vi "Execute Single Statement (String Parameters).vi"(6 "Oids":i32[](array[numeric]), 8 "error in (no error)":errorcluster, 9 "Parameters":string[](array[string]), 10 "SQL (Single Command)":string, 11 "PQ Connection in":refnum<class "PQ Connection.lvclass">) -> (0 "error out":errorcluster, 1 "First Result with Rows returned":refnum<class "PQ Result.lvclass">, 2 "Number of Rows":i32, 3 "PQ Connection out":refnum<class "PQ Connection.lvclass">)   [LabVIEW 2013, in "PQ Connection.lvclass"]
uses:
  PQ Connection.lvclass
  Result/PQ Result.lvclass
  PQ Connection.lvclass/PQ Connection.ctl
  Result/PQ Result.lvclass/PQ Result.ctl
  Support/PQ Support.lvlib
  libpq.dll
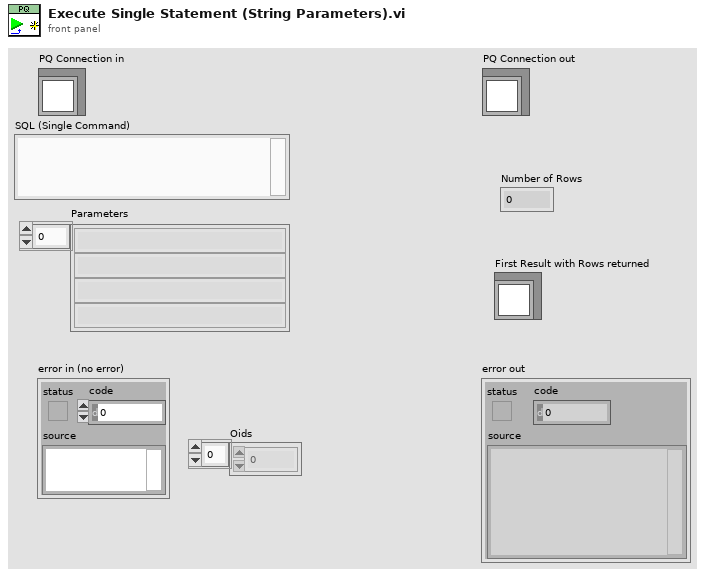
[diagram p1: front panel]
types:
  T1 = typedef "PQ Result.lvclass/Result Status.ctl" = enum32{"PGRES_EMPTY_QUERY", "PGRES_COMMAND_OK", "PGRES_TUPLES_OK", "PGRES_COPY_OUT", "PGRES_COPY_IN", "PGRES_BAD_RESPONSE", "PGRES_NONFATAL_ERROR", "PGRES_FATAL_ERROR", "PGRES_COPY_BOTH", "PGRES_SINGLE_TUPLE"}
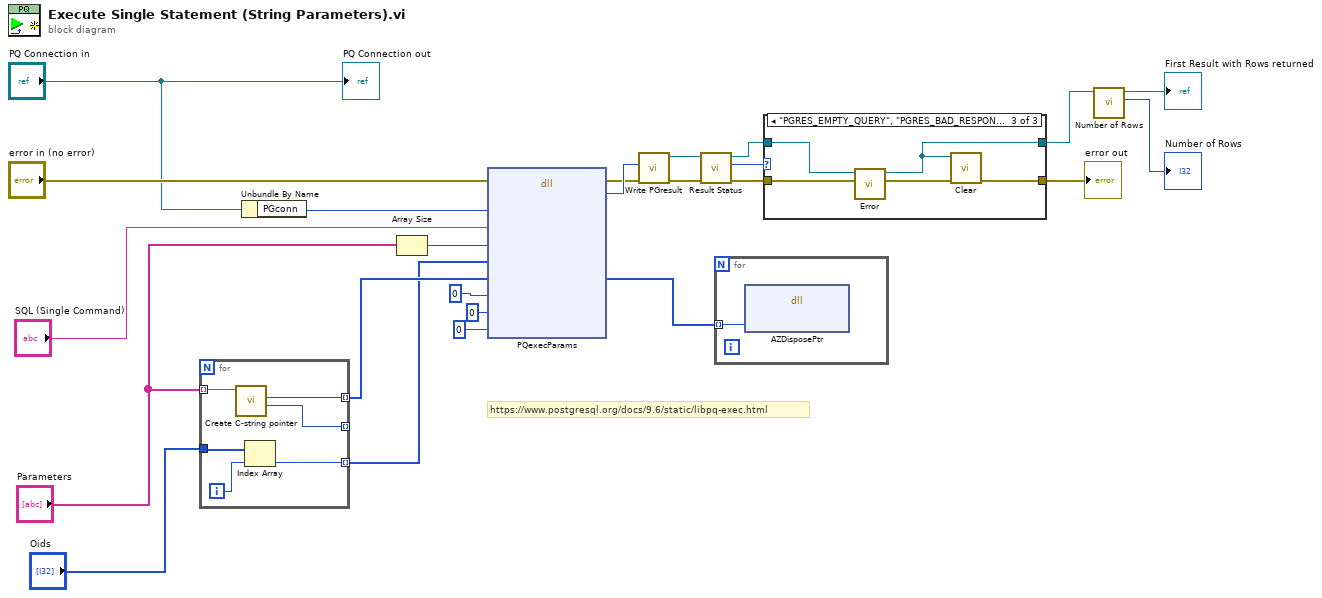
[diagram p0: block diagram]
diagram:
  # "https://www.postgresql.org/docs/9.6/static/libpq-exec.html"
  n1 = for {
    tunnel: "Parameters" -> [w30] mode=indexing
    tunnel: [w29] -> w7 mode=indexing
    tunnel: [w28] -> _ mode=indexing
    tunnel: "Oids" -> [w27]
    tunnel: [w25] -> w1 mode=indexing
    i -> [w26]
    n2 = call "Create C-string pointer.vi"("string"=w30) -> ("size"=w28:i32, "C-string pointer"=w29:i64)  [unwired: 7 in, 2 out]
    n3 = Index Array(array=w27, index=w26) -> (element=w25:i32)
  }
  n4 = Unbundle By Name("PQ Connection in") -> ("PGconn"=w23:u32)
  n5 = Array Size(array="Parameters") -> (size(s)=w9:i32)
  n6 = dll-call lib="C:/Users/patrick/Documents/GitHub/DSC/src/PostgreSQL Library/Connection/libpq.dll" fn="PQexecParams" ("libpq.*:PQexec")(error in="error in (no error)", "PGconn"=w23, "command"="SQL (Single Command)", "nParams"=w9, "Types"=w1, "Values"=w7, "Lengths"=0 ("Types"), "Formats"=0, "Result Format"=0) -> (error out=w10:errorcluster, "PQresult"=w11:u32, "Values"=w5:i64[])  [unwired: 9 in, 1 out]
  n7 = call "Write PGresult.vi"("error in (no error)"=w10, "PGresult"=w11) -> ("error out"=w15:errorcluster, "PQ Result  out"=w16:refnum<class "PQ Result.lvclass">)  [unwired: 8 in]
  n8 = call "Result Status.vi"("error in (no error)"=w15, "PQ Result in"=w16) -> ("error out"=w12:errorcluster, "Result Status"=w14:T1, "PQ Result out"=w13:refnum<class "PQ Result.lvclass">)  [unwired: 7 in]
  n9 = for {
    tunnel: w5 -> [w31] mode=indexing
    n10 = dll-call lib="LabVIEW" fn="AZDisposePtr"("pointer"=w31) -> ()  [unwired: 5 in, 2 out]
  }
  n11 = case shown="\"PGRES_EMPTY_QUERY\", \"PGRES_BAD_RESPONSE\", \"PGRES_FATAL_ERROR\"" w14 {
    tunnel: [w32 w34 w38] -> w18
    tunnel: w13 -> [w32 w34 w40]
    tunnel: w12 -> [w33 w35 w39]
    tunnel: [w33 w35 w36] -> w17
    frame "PGRES_TUPLES_OK" {
    }
    frame Default {
      # "No results, but not error"
    }
    frame "PGRES_EMPTY_QUERY", "PGRES_BAD_RESPONSE", "PGRES_FATAL_ERROR" {
      n12 = call "Error.vi"("error in (no error)"=w39, "PQ Result  In"=w40) -> ("error out"=w37:errorcluster, "PQ Result"=w38:refnum<class "PQ Result.lvclass">)  [unwired: 8 in]
      n13 = call "Clear.vi"("error in (no error)"=w37, "PQ Result  in"=w38) -> ("error out"=w36:errorcluster)  [unwired: 9 in]
    }
  }
  "error out" <- w17
  n14 = call "Number of Rows.vi"("PQ Result in"=w18) -> ("Number of Rows"=→"Number of Rows":i32, "PQ Result out"=→"First Result with Rows returned":refnum<class "PQ Result.lvclass">)  [unwired: 8 in, 1 out]
  "PQ Connection out" <- "PQ Connection in"
